vi "FTW-JSON-CompareEquality.vi"(0 "JSON Object":refnum<class "FTW-JSON.lvclass">, 5 "JSON Object to Compare":refnum<class "FTW-JSON.lvclass">, 11 "error in":errorcluster) -> (4 "Equal?":bool, 15 "error out":errorcluster)   [LabVIEW 2013, in "FTW-JSON.lvclass"]
uses:
  FTW-JSON.lvclass
  FTW-JSON.lvclass/FTW-JSON.ctl
panel:
  # "Inputs"
  # "Outputs"
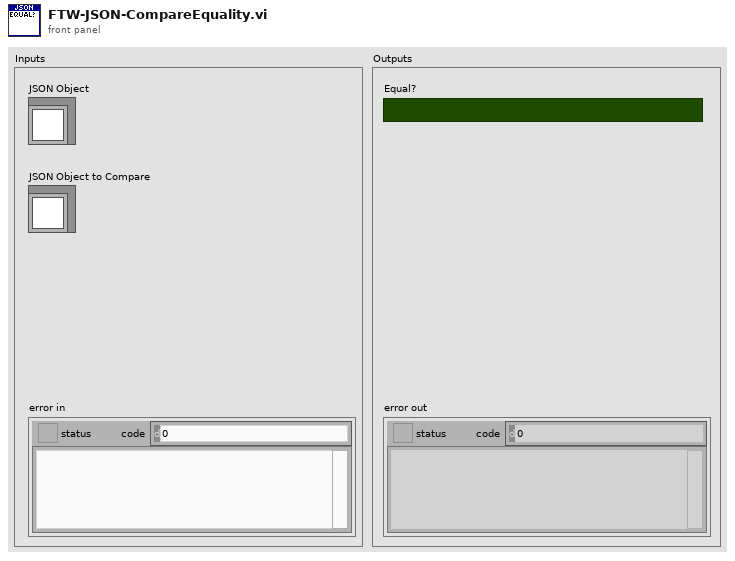
[diagram p1: front panel]
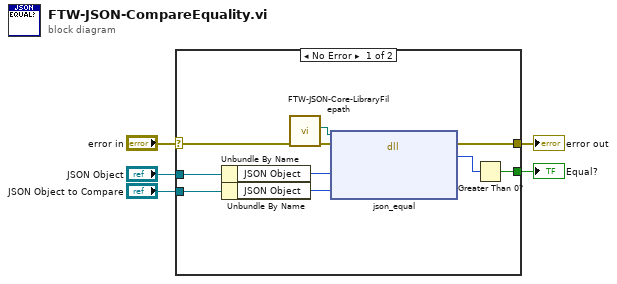
[diagram p0: block diagram]
diagram:
  n1 = case shown="No Error" "error in" {
    selector: "error in" -> [w15 w16]
    tunnel: [w14 w16] -> w5
    tunnel: "JSON Object" -> [w13 _]
    tunnel: [w8 _] -> w2
    tunnel: "JSON Object to Compare" -> [w7 _]
    frame No Error {
      n2 = Unbundle By Name(w13) -> ("JSON Object"=w9:i64)
      n3 = Unbundle By Name(w7) -> ("JSON Object"=w6:i64)
      n4 = call "FTW-JSON-Core-LibraryFilepath.vi"("error in"=w15) -> ("error out"=w11:errorcluster, "JSON Library Filepath"=w10:path)  [unwired: 9 in]
      n5 = dll-call lib="?" fn="json_equal"(path in=w10, error in=w11, "JSON Object Pointer 1"=w9, "JSON Object Pointer 2"=w6) -> (error out=w14:errorcluster, "Are Objects Equal?"=w12:u8)  [unwired: 3 in, 1 out]
      n6 = Greater Than 0?(x=w12) -> (x > 0?=w8:bool)
    }
    frame Error {
    }
  }
  "error out" <- w5
  "Equal?" <- w2
